vi "PH_PPPA_PowerUnit.src Wait for Shot Cmd.vi"(0 "i ref in":refnum<vi>, 5 "error in (no error)":errorcluster) -> (14 "i ref out":refnum<vi>, 19 "error out":errorcluster)   [LabVIEW 2014, in "PH_PPPA_PowerUnit.lvlib"]
doc: "This is the action VI of the Shot event case. It checks the state of the SM and related Devices. If\n\nState SM = \"Wait for Shot Cmd\",\nWaiting Time over? = true,\nState RR = false (closed), \nState PSU = off, \nIgnitron.State Device = on, and\nPPPA PU State = Running,\n\nthen a request state change is send to the SM to get \"Open Ross Relais\"."
uses:
  PH_PPPA_PowerUnit.lvlib
  PH_StatusHandler/PH_StatusHandler.Status.ctl
  PH_PowerUnit_BaseClass/PH_PowerUnit_BaseClass.SM States.ctl
  PH_StatusHandler/PH_StatusHandler.lvlib
  PH_PowerUnit_BaseClass/PH_PowerUnit_BaseClass.lvlib
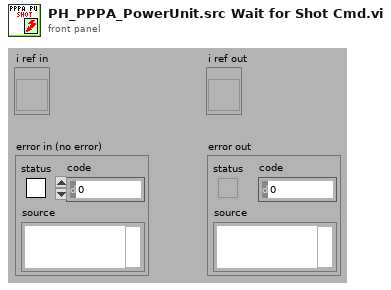
[diagram p1: front panel]
types:
  T1 = typedef "PH_PowerUnit_BaseClass.lvlib/PH_PowerUnit_BaseClass.SM States.ctl" = enum16{".", "Stand by", "Switch PU on", "Configure", "Set Default Voltage", "Set STANDBY", "Set READY", "Wait for Shot Cmd", "Open Dump Rods", "Open Ross Relais", "Close Ross Relais", "Switch PSU on", "Switch PSU off", "Charge", "Switch GD Channel on", "Close Dump Rods", "Rods-TO", "RR-TO", "PSU-TO", "Trigger-TO"}
  T2 = typedef "PH_StatusHandler.lvlib/PH_StatusHandler.Status.ctl" = i16
  T3 = typedef "PH_PowerUnit_BaseClass.lvlib/PH_PowerUnit_BaseClass.i attribute.ctl" = cluster{"Constructor finished":bool, "PU":cluster{"In use":bool, "Service ID in use":i32, "GUI Ref":refnum<vi>}, "Enabling":cluster{"State":T4, "GUI Ref":refnum<vi>}, "Timing":cluster{"Last Shot":dbl, "Time between Shots [Sec]":dbl, "Waiting Time over?":bool, "Service ID Waiting Time":i32, "GUI Ref":refnum<vi>, "Instance":cluster{"Status":T2, "linked?":bool, "GUI Ref":refnum<vi>}}, "Sequencer":cluster{"SM State":string, "GUI Ref":refnum<vi>, "linked":bool}, "Subscribed Trendmssgs":cluster{"Tagname":string, "Status":T2, "linked?":bool, "Shot Condition":T2, "GUI Ref":refnum<vi>}[], "PP PU":T5, "Default Voltage (V)":dbl, "GUI Refs":T6, "PSDB data":cluster{"Shot Voltage [V]":dbl, "State TO SM":T1, "Write 2 early":bool}, "State TO SM":T1}
  T4 = typedef "PH_SystemInformation.lvlib/PH_SystemInformationEnabling State.ctl" = i32
  T5 = typedef "PH_PP_Common.lvlib/PH_PP_Common.PUs.ctl" = enum16{"no Info", "PA-19mm-1", "PA-19mm-2", "PA-45mm-PILC", "PA-45mm-MAIN", "MA-PU-1", "MA-PU-2", "MA-PU-3", "MA-PU-4", "MA-PU-5", "MA-PU-6", "MA-FR", "MA-PILC", "PA-45mm-DP"}
  T6 = typedef "PH_PowerUnit_BaseClass.lvlib/PH_PowerUnit_BaseClass.GUI Refs.ctl" = cluster{"Delete Inst":refnum<vi>, "State TO SM":refnum<vi>, "State SM":refnum<vi>, "Fire":refnum<vi>}
  T7 = typedef "PH_PPPA_PowerUnit.lvlib/PH_PPPA_PowerUnit.i attribute.ctl" = cluster{"GUI Refs":cluster{"Ignitron":refnum<vi>, "Rossrelais":refnum<vi>, "Set Voltage":refnum<vi>, "PSU":refnum<vi>, "EOC":refnum<vi>, "Trigger":refnum<vi>}, "Ignitron":T8, "PSU":T9, "Dump Ross Relais":T10, "Trigger":cluster{"State Device":T2, "linked?":bool}, "Timing Settings":cluster{"Prdc Fast?":bool, "Default Value Periodic Interval":i32, "Mercury on since":dbl, "Warm up Time Mercury [s]":dbl}, "Set Voltage [V]":dbl, "19er Ignitionbox":string}
  T8 = typedef "PH_PP_Common.lvlib/PH_PP_Common.Ignitron Attributes.ctl" = cluster{"State Device":T2, "linked?":bool}
  T9 = typedef "PH_PP_Common.lvlib/PH_PP_Common.PSU Attributes.ctl" = cluster{"lower limit [V]":dbl, "upper limit [V]":dbl, "Voltage set":bool, "State Device":T2, "linked?":bool}
  T10 = typedef "PH_PP_Common.lvlib/PH_PP_Common.Ross Relais Attributes.ctl" = cluster{"State Device":T2, "linked?":bool}
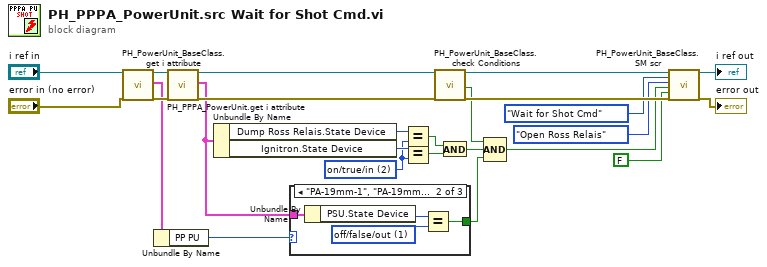
[diagram p0: block diagram]
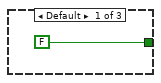
[diagram p2: hidden frame]
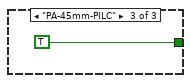
[diagram p3: hidden frame]
diagram:
  w11 = T2 2 items=["no info", "off/false/out", "on/true/in", "Failure", "Alarm", "Status 1", "Status 2", "Status 3"] ("Dump Ross Relais.State Device")
  n1 = call "PH_PowerUnit_BaseClass.get i attribute.vi"("i ref in"="i ref in", "error in (no error)"="error in (no error)") -> ("i ref out"=w20:refnum<vi>, "i attribute"=w8:T3, "error out"=w22:errorcluster)  [unwired: 15 in]
  n2 = Unbundle By Name(w8) -> ("PP PU"=w7:T5)
  n3 = call "PH_PPPA_PowerUnit.get i attribute.vi"("i ref in"=w20, "error in (no error)"=w22) -> ("i ref out"=w18:refnum<vi>, "i attribute"=w10:T7, "error out"=w25:errorcluster)  [unwired: 15 in]
  n4 = Unbundle By Name(w10) -> ("Dump Ross Relais.State Device"=w15:T2, "Ignitron.State Device"=w13:T2)
  n5 = case shown="\"PA-19mm-1\", \"PA-19mm-2\", \"PA-45mm-MAIN\"" w7 {
    tunnel: w10 -> [_ w30 _]
    tunnel: [FALSE w27 TRUE] -> w23
    frame Default {
    }
    frame "PA-19mm-1", "PA-19mm-2", "PA-45mm-MAIN" {
      w28 = T2 1 items=["no info", "off/false/out", "on/true/in", "Failure", "Alarm", "Status 1", "Status 2", "Status 3"] ("Dump Ross Relais.State Device")
      n6 = Unbundle By Name(w30) -> ("PSU.State Device"=w29:T2)
      n7 = Equal?(x=w29, y=w28) -> (x = y?=w27:bool)
    }
    frame "PA-45mm-PILC" {
    }
  }
  n8 = Equal?(x=w15, y=w11) -> (x = y?=w14:bool)
  n9 = Equal?(x=w13, y=w11) -> (x = y?=w12:bool)
  n10 = call "PH_PowerUnit_BaseClass.check Conditions.vi"("VI in"=w18, "error in (no error)"=w25) -> ("VI out"=w17:refnum<vi>, "Ready for shot"=w16:bool, "error out"=w19:errorcluster)  [unwired: 14 in, 1 out]
  n11 = And(x=w14, y=w12) -> (x .and. y?=w9:bool)
  n12 = Compound Arithmetic op=AND(w16, w9, w23) -> (w6:bool)
  n13 = call "PH_PowerUnit_BaseClass.SM scr.vi"("VI in"=w17, "Current SM State (condition)"=PH_PowerUnit_BaseClass.SM_States."Wait for Shot Cmd", "Wanted SM State"=PH_PowerUnit_BaseClass.SM_States."Open Ross Relais", "Further change condition"=w6, "PU in use is condition? (true)"=FALSE, "error in (no error)"=w19) -> ("VI out"=→"i ref out":refnum<vi>, "error out"=→"error out":errorcluster)  [unwired: 12 in]
